vi "E14 BBB Test.vi"(8 "Error In":errorcluster, 11 "Install LV Data":T1={"SSH Session"=refnum, "Status Log"="", "Detailed Log"="", "Credentials"={"Hostname or IP"="192.168.7.2", "Username"="root", "Password"=""}, "Target Info"={"OS Version"="", "CPU"="", "Systemd Version"="", "Internet Access"=FALSE, "Device Type"="", "LV Installed Ver"="", "LV Available Ver"="", "LV Upgrade Available"=FALSE, "Hostname"="", "NIC Info"=[]}, "Reboot Required?"=FALSE}) -> (0 "Error Out":errorcluster, 1 "Status":string, 3 "Install LV Data":T1={"SSH Session"=refnum, "Status Log"="", "Detailed Log"="", "Credentials"={"Hostname or IP"="192.168.7.2", "Username"="root", "Password"=""}, "Target Info"={"OS Version"="", "CPU"="", "Systemd Version"="", "Internet Access"=FALSE, "Device Type"="", "LV Installed Ver"="", "LV Available Ver"="", "LV Upgrade Available"=FALSE, "Hostname"="", "NIC Info"=[]}, "Reboot Required?"=FALSE})   [LabVIEW 2014, in "LMH-LINX.lvlib"]
uses:
  <vilib>/MakerHub/LINX/LMH-LINX.lvlib
  <vilib>/MakerHub/LINX/Private/Utilties/Target Management/Install LV Data.ctl
  C:/Program Files (x86)/National Instruments/LabVIEW 2014/vi.lib/MakerHub/LINX/Resources/Renci.SshNet.dll
  Resources/Renci.SshNet.dll
  <vilib>/MakerHub/LINX/Private/Utilties/Target Management/Target Info.ctl
  <vilib>/MakerHub/LINX/Private/Utilties/Target Management/NIC Info.ctl
  <vilib>/MakerHub/LINX/Private/Utilties/Target Management/NIC Mode.ctl
  <vilib>/MakerHub/Toolbox/LMH-Toolbox.lvlib
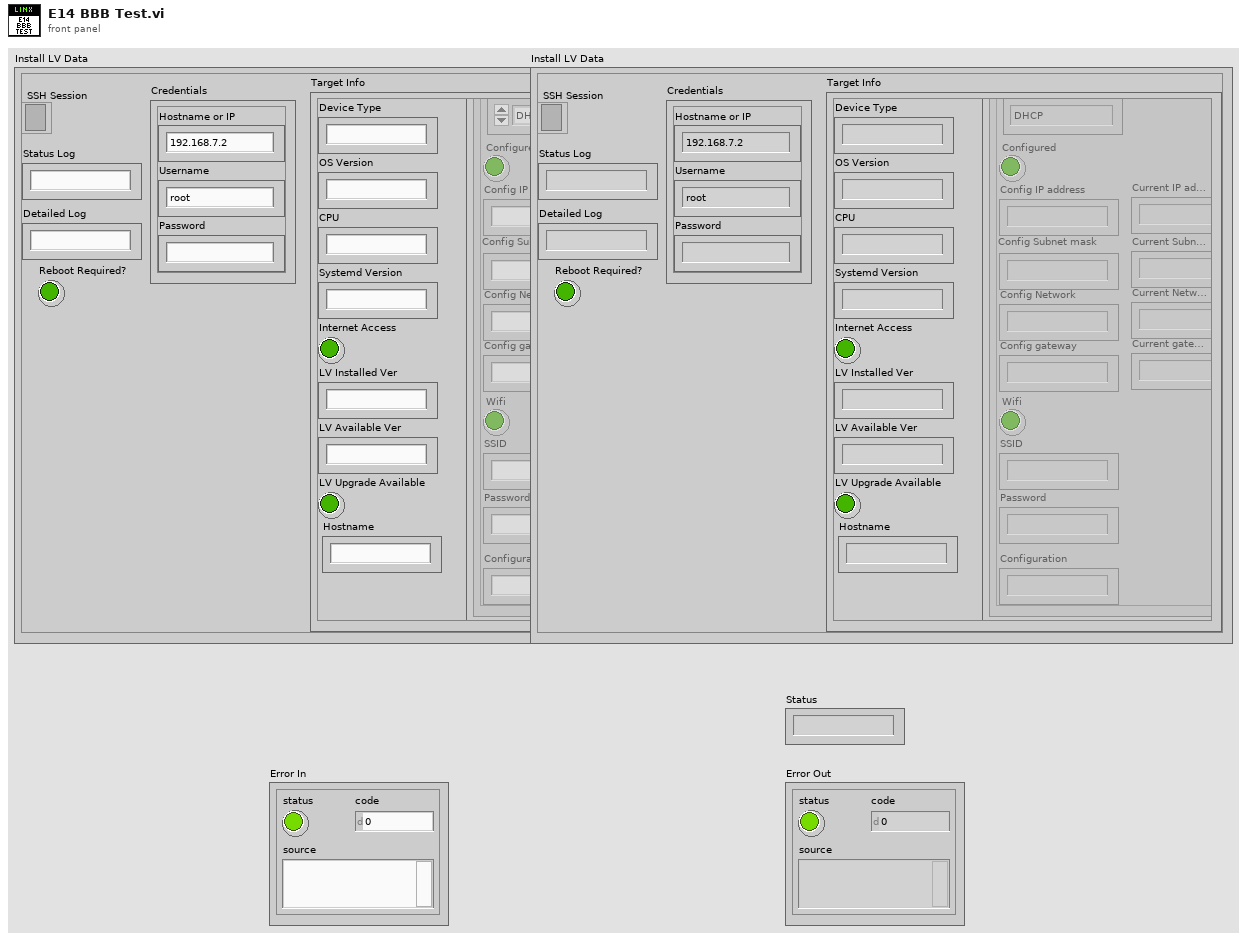
[diagram p1: front panel]
types:
  T1 = typedef "LMH-LINX.lvlib/Install LV Data.ctl" = cluster{"SSH Session":refnum<k24>, "Status Log":string, "Detailed Log":string, "Credentials":cluster{"Hostname or IP":string, "Username":string, "Password":string}, "Target Info":T2, "Reboot Required?":bool}
  T2 = typedef "LMH-LINX.lvlib/Target Info.ctl" = cluster{"OS Version":string, "CPU":string, "Systemd Version":string, "Internet Access":bool, "Device Type":string, "LV Installed Ver":string, "LV Available Ver":string, "LV Upgrade Available":bool, "Hostname":string, "NIC Info":T3[]}
  T3 = typedef "LMH-LINX.lvlib/NIC Info.ctl" = cluster{"Name":string, "NIC Mode":T4, "Configured":bool, "Config IP address":string, "Config Subnet mask":string, "Config Network":string, "Config gateway":string, "Wifi":bool, "SSID":string, "Password":string, "Configuration":string, "Current IP address":string, "Current Subnet mask":string, "Current gateway":string, "Current Network":string}
  T4 = typedef "LMH-LINX.lvlib/NIC Mode.ctl" = enum16{"DHCP", "Static", "Loopback"}
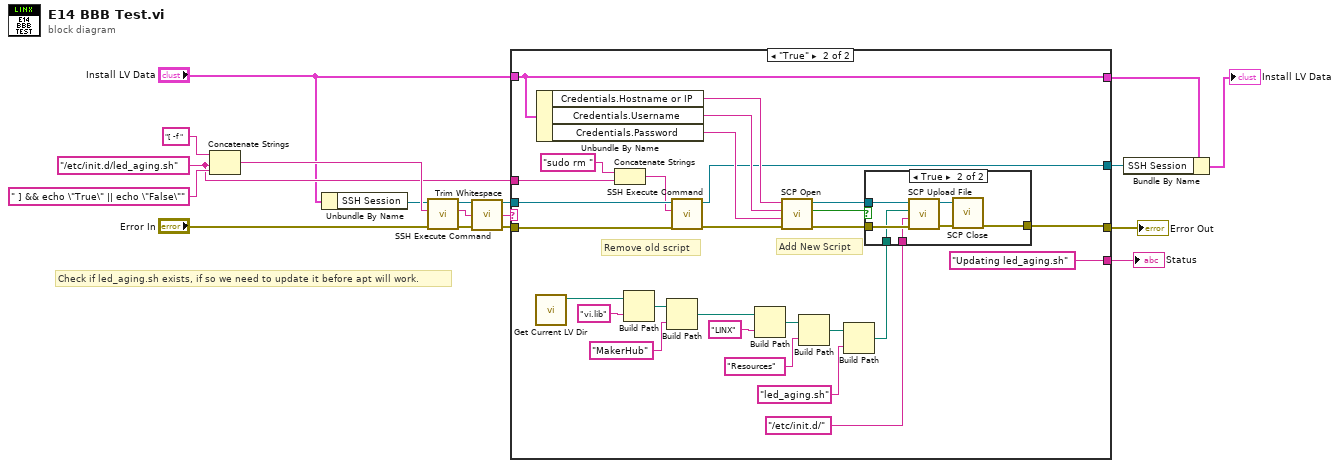
[diagram p0: block diagram]
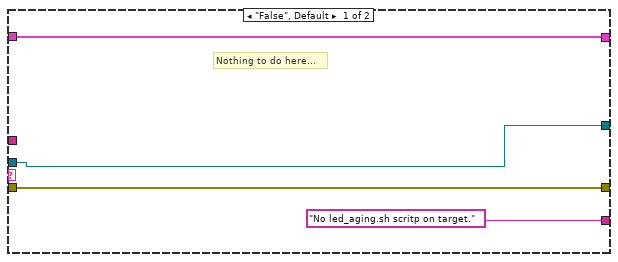
[diagram p2: hidden frame]
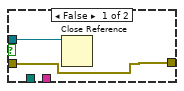
[diagram p3: hidden frame]
diagram:
  w10 = "/etc/init.d/led_aging.sh" ("Command")
  # "Check if led_aging.sh exists, if so we need to update it before apt will work."
  n1 = Concatenate Strings("[ -f " ("Command"), w10, " ] && echo \"True\" || echo \"False\"" ("Command")) -> (w11:string)
  n2 = Unbundle By Name("Install LV Data") -> ("SSH Session"=w6:refnum<k24>)
  n3 = call <vilib>:"SSH Execute Command.vi"("Error In"="Error In", "Command"=w11, "SSH Session"=w6) -> ("Error Out"=w15:errorcluster, "Std Out"=w8:string, "SSH Session"=w14:refnum<k24>)  [unwired: 6 in]
  n4 = call <vilib>:"Trim Whitespace.vi"("string"=w8) -> ("trimmed string"=w7:string)  [unwired: 1 in]
  n5 = case shown="\"True\"" w7 {
    tunnel: w15 -> [w20 w48]
    tunnel: w14 -> [w18 w47]
    tunnel: w10 -> [_ w44]
    tunnel: [w20 w25] -> w9
    tunnel: "Install LV Data" -> [w17 w22]
    tunnel: [w17 w22] -> w1
    tunnel: ["No led_aging.sh scritp on target." ("Std Out") "Updating led_aging.sh" ("Std Out")] -> w4
    tunnel: [w18 w23] -> w3
    frame "False", Default {
      # "Nothing to do here..."
    }
    frame "True" {
      # "Remove old script"
      # "Add New Script"
      n6 = call <vilib>:"Get Current LV Dir.vi"() -> ("This LV Directory"=w28:path)  [unwired: 10 in, 1 out]
      n7 = Unbundle By Name(w22) -> ("Credentials.Hostname or IP"=w43:string, "Credentials.Username"=w42:string, "Credentials.Password"=w40:string)
      n8 = Concatenate Strings("sudo rm " ("Command"), w44) -> (w45:string)
      n9 = Build Path(base path=w28, name or relative path="vi.lib" ("Command")) -> (appended path=w30:path)
      n10 = Build Path(base path=w30, name or relative path="MakerHub" ("Command")) -> (appended path=w31:path)
      n11 = call <vilib>:"SSH Execute Command.vi"("Error In"=w48, "Command"=w45, "SSH Session"=w47) -> ("Error Out"=w41:errorcluster, "SSH Session"=w23:refnum<k24>)  [unwired: 6 in, 1 out]
      n12 = Build Path(base path=w31, name or relative path="LINX" ("Command")) -> (appended path=w32:path)
      n13 = call <vilib>:"SCP Open.vi"("Error In"=w41, "Password"=w40, "Username"=w42, "Hostname or IP"=w43) -> ("Error Out"=w38:errorcluster, "Connected?"=w24:bool, "SCP Session"=w39:refnum<k24>)  [unwired: 5 in]
      n14 = Build Path(base path=w32, name or relative path="Resources" ("Command")) -> (appended path=w37:path)
      n15 = Build Path(base path=w37, name or relative path="led_aging.sh") -> (appended path=w27:path)
      n16 = case shown="True" w24 {
        tunnel: w39 -> [w50 w57]
        tunnel: w38 -> [w49 w56]
        tunnel: w27 -> [_ w55]
        tunnel: "/etc/init.d/" ("Target Directory") -> [_ w52]
        tunnel: [w49 w51] -> w25
        frame False {
          n17 = Close Reference(reference=w50) -> ()  [unwired: 1 in, 1 out]
        }
        frame True {
          n18 = call <vilib>:"SCP Upload File.vi"("Error In"=w56, "Target Directory"=w52, "Local File"=w55, "SCP Session"=w57) -> ("Error Out"=w53:errorcluster, "SCP Session"=w54:refnum<k24>)  [unwired: 6 in]
          n19 = call <vilib>:"SCP Close.vi"("Error In"=w53, "SCP Session"=w54) -> ("Error Out"=w51:errorcluster)  [unwired: 9 in]
        }
      }
    }
  }
  "Error Out" <- w9
  "Status" <- w4
  n20 = Bundle By Name(cluster=w1, "SSH Session"=w3) -> (→"Install LV Data":T1)
